vi "CombineMoveSegments.vi"(1 "Path":T3) -> (0 "Combined Moves (Discarding Metadata Save Moved Fwd)":T1[](array[typedef]))   [LabVIEW 2015]
doc: "Combines moves in a path that head in same direction. Discards a bunch of other info about moves, as this is just a convenience function used when moving the bot along the path."
uses:
  Computer_VIs/PathOfMoves.ctl
  Computer_VIs/Move.ctl
  Computer_VIs/Vector.ctl
  Computer_VIs/Navigation2017.lvlib
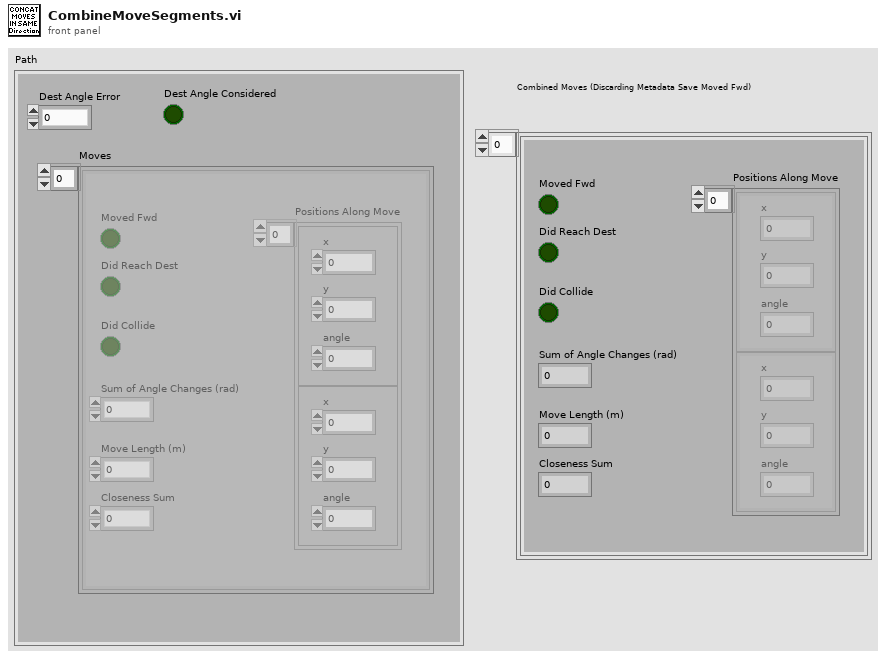
[diagram p1: front panel]
types:
  T1 = typedef "Navigation2017.lvlib/Move.ctl" = cluster{"Did Reach Dest":bool, "Did Collide":bool, "Sum of Angle Changes (rad)":dbl, "Move Length (m)":dbl, "Closeness Sum":dbl, "Positions Along Move":T2[], "Moved Fwd":bool}
  T2 = typedef "Navigation2017.lvlib/Vector.ctl" = cluster{"x":dbl, "y":dbl, "angle":dbl}
  T3 = typedef "Navigation2017.lvlib/PathOfMoves.ctl" = cluster{"Dest Angle Error":dbl, "Dest Angle Considered":bool, "Moves":T1[]}
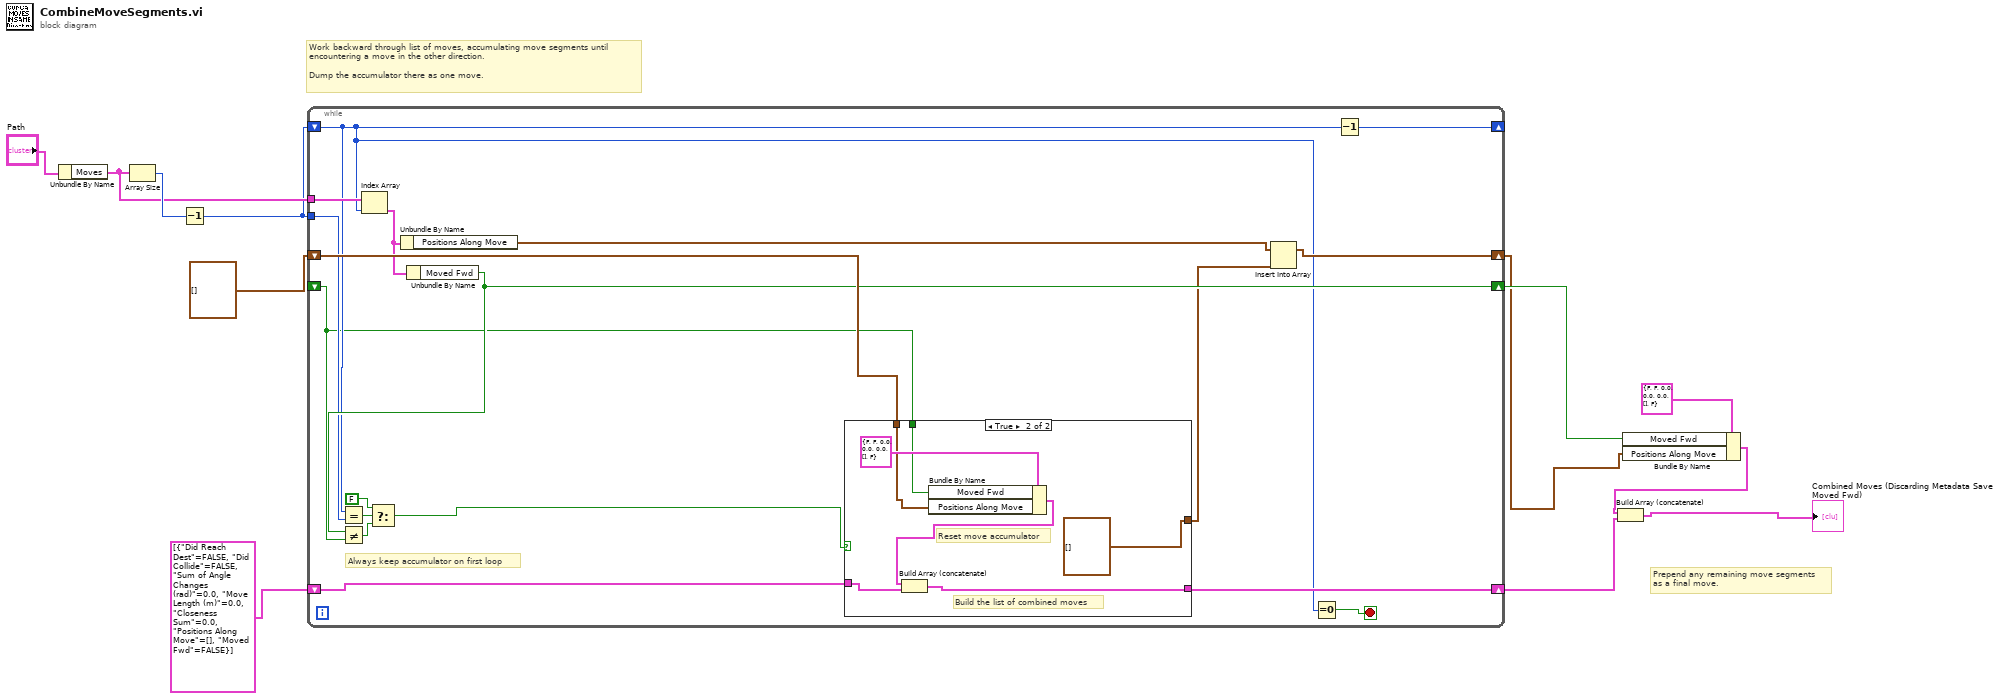
[diagram p0: block diagram]
diagram:
  # "Prepend any remaining move segments\nas a final move."
  # "Work backward through list of moves, accumulating move segments until\nencountering a move in the other direction. \n\nDump the accumulator there as one move."
  n1 = Unbundle By Name("Path") -> ("Moves"=w11:T1[])
  n2 = Array Size(array=w11) -> (size(s)=w12:i32)
  n3 = Decrement(x=w12) -> (x-1=w9:i32)
  n4 = while {
    shift-right: [w30] -> _
    shift-left: w9 -> [w17]
    shift-right: [w29] -> w8
    shift-left: T1[] [{"Did Reach Dest"=FALSE, "Did Collide"=FALSE, "Sum of Angle Changes (rad)"=0.0, "Move Length (m)"=0.0, "Closeness Sum"=0.0, "Positions Along Move"=[], "Moved Fwd"=FALSE}] -> [w28]
    tunnel: w11 -> [w27]
    shift-right: [w25] -> w3
    shift-left: T2[] [] -> [w26]
    shift-right: [w24] -> w4
    shift-left: _ -> [w13]
    tunnel: w9 -> [w22]
    stop <- w18 stop-if-true
    # "Always keep accumulator on first loop"
    n5 = Equal?(x=w17, y=w22) -> (x = y?=w23:bool)
    n6 = Index Array(array=w27, index=w17) -> (element=w14:T1)
    n7 = Unbundle By Name(w14) -> ("Positions Along Move"=w16:T2[])
    n8 = Unbundle By Name(w14) -> ("Moved Fwd"=w24:bool)
    n9 = Not Equal?(x=w24, y=w13) -> (x != y?=w20:bool)
    n10 = Select(t=FALSE, s=w23, f=w20) -> (s? t:f=w19:bool)
    n11 = case shown="True" w19 {
      tunnel: [w31 w39] -> w29
      tunnel: w28 -> [w31 w37]
      tunnel: w26 -> [w32 w34]
      tunnel: [w32 T2[] []] -> w15
      tunnel: w13 -> [_ w35]
      frame False {
      }
      frame True {
        # "Reset move accumulator"
        # "Build the list of combined moves"
        n12 = Bundle By Name(cluster=T1 {"Did Reach Dest"=FALSE, "Did Collide"=FALSE, "Sum of Angle Changes (rad)"=0.0, "Move Length (m)"=0.0, "Closeness Sum"=0.0, "Positions Along Move"=[], "Moved Fwd"=FALSE} ("Move"), "Moved Fwd"=w35, "Positions Along Move"=w34) -> (w33:T1)
        n13 = Build Array (concatenate)(w33, w37) -> (w39:T1[])
      }
    }
    n14 = Insert Into Array(array=w16, new element=w15) -> (w25:T2[])  [unwired: 1 in]
    n15 = Equal To 0?(x=w17) -> (x = 0?=w18:bool)
    n16 = Decrement(x=w17) -> (x-1=w30:i32)
  }
  n17 = Bundle By Name(cluster=T1 {"Did Reach Dest"=FALSE, "Did Collide"=FALSE, "Sum of Angle Changes (rad)"=0.0, "Move Length (m)"=0.0, "Closeness Sum"=0.0, "Positions Along Move"=[], "Moved Fwd"=FALSE} ("Move"), "Moved Fwd"=w4, "Positions Along Move"=w3) -> (w2:T1)
  n18 = Build Array (concatenate)(w2, w8) -> (→"Combined Moves (Discarding Metadata Save Moved Fwd)":T1[])
